vi "_PC_Daemon_Laser_CheckEmission.vi"(1 "stopRefnum":refnum<vi>, 2 "error in (no error)":errorcluster, 3 "LaserSetting":T1={"Energy"=50.0, "Freq"=100.0, "Emission"=FALSE, "TriggerSource"=enum."Internal", "Time Stamp"=timestamp(0 s since 1904-01-01)}) -> (0 "error out":errorcluster)   [LabVIEW 2018]
uses:
  RT/ControlLoop/Laser/Ctl/_ctl_LaserParam.ctl
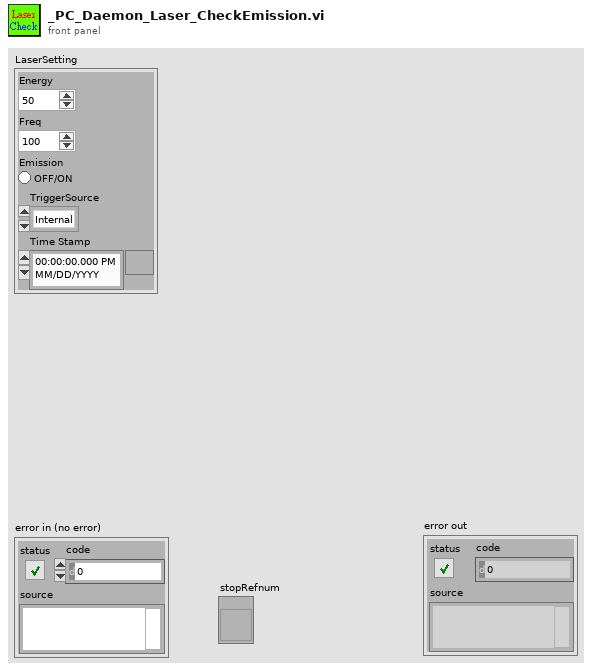
[diagram p1: front panel]
types:
  T1 = typedef "_ctl_LaserParam.ctl" = cluster{"Energy":dbl, "Freq":dbl, "Emission":bool, "TriggerSource":enum16{"Internal", "External"}, "Time Stamp":timestamp}
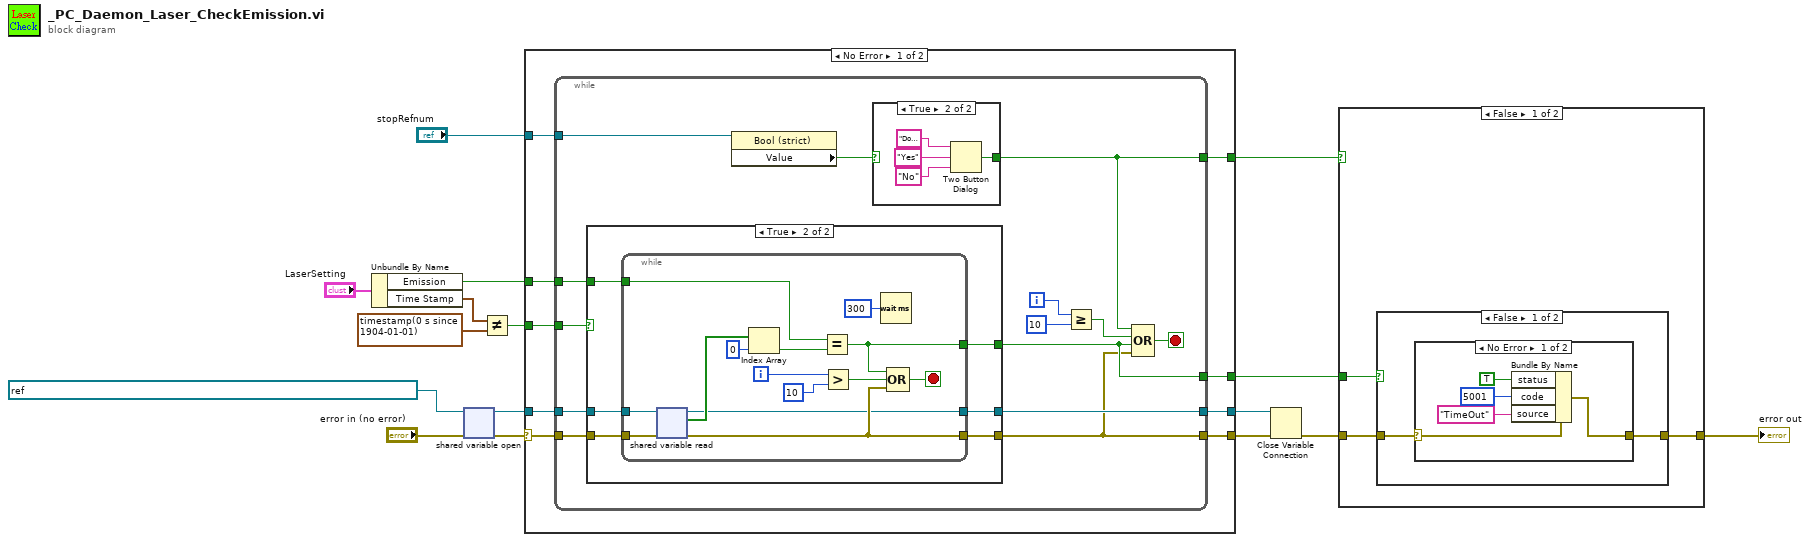
[diagram p0: block diagram]
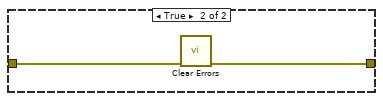
[diagram p4: hidden frame]
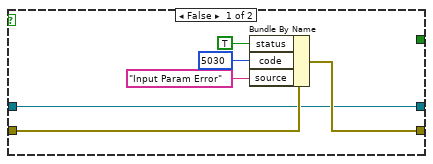
[diagram p6: hidden frame]
diagram:
  n1 = Unbundle By Name("LaserSetting") -> ("Emission"=w14:bool, "Time Stamp"=w16:timestamp)
  n2 = shared-variable-open(refnum<k21> "ni.var.psp://NI-sbRIO/_RT_CtrlLoop_Laser_Variables/LaserStatusByte" ("shared variable refnum in"), "error in (no error)") -> (w7:refnum<k21>, w6:errorcluster)
  n3 = Not Equal?(x=w16, y=timestamp(0 s since 1904-01-01)) -> (x != y?=w13:bool)
  n4 = case shown="No Error" w6 {
    selector: w6 -> [w20 w72]
    tunnel: w14 -> [w25 _]
    tunnel: w13 -> [w24 _]
    tunnel: [w23 w72] -> w4
    tunnel: [w22 _] -> w11
    tunnel: w7 -> [w21 w71]
    tunnel: [w19 w71] -> w5
    tunnel: "stopRefnum" -> [w18 _]
    tunnel: [w17 _] -> w1
    frame No Error {
      n5 = while {
        tunnel: w25 -> [w39]
        tunnel: w24 -> [w38]
        tunnel: [w29] -> w23
        tunnel: [w33] -> w22
        tunnel: w21 -> [w32]
        tunnel: w20 -> [w31]
        tunnel: [w30] -> w19
        tunnel: w18 -> [w28]
        tunnel: [w26] -> w17
        i -> [w37]
        stop <- w34 stop-if-true
        n6 = case shown="True" w38 {
          tunnel: w39 -> [_ w56]
          tunnel: [_ w55] -> w33
          tunnel: w32 -> [w45 w54]
          tunnel: w31 -> [w47 w53]
          tunnel: [w46 w52] -> w29
          tunnel: [w45 w51] -> w30
          frame False {
            n7 = Bundle By Name(cluster=w47, "status"=TRUE, "code"=5030, "source"="Input Param Error") -> (w46:errorcluster)
          }
          frame True {
            n8 = while {
              tunnel: w56 -> [w66]
              tunnel: [w63] -> w55
              tunnel: w54 -> [w62]
              tunnel: w53 -> [w61]
              tunnel: [w58] -> w52
              tunnel: [w57] -> w51
              i -> [w65]
              stop <- w67 stop-if-true
              n9 = shared-variable-read(w62, w61) -> (w57:refnum<k21>, w58:errorcluster, w60:bool[])
              n10 = Index Array(array=w60, index=0) -> (element=w69:bool)
              n11 = Equal?(x=w66, y=w69) -> (x = y?=w63:bool)
              n12 = Greater?(x=w65, y=10) -> (0:w59:bool)
              n13 = Wait (ms)(milliseconds to wait=u32 300) -> ()  [unwired: 1 out]
              n14 = Compound Arithmetic op=OR(w63, w59, w58) -> (w67:bool)
            }
          }
        }
        n15 = property class="Bool (strict)"(reference=w28) -> ("Value"=w27:bool)  [unwired: 1 in, 2 out]
        n16 = case shown="True" w27 {
          selector: w27 -> [w40 _]
          tunnel: [w40 w41] -> w26
          frame False {
          }
          frame True {
            n17 = Two Button Dialog(message="Do you want to confirm the interrupt in the parameter setting?", 1:"No" ("F button name (\"Cancel\")"), 2:"Yes" ("T button name (\"OK\")")) -> (T button?=w41:bool)
          }
        }
        n18 = Greater Or Equal?(x=w37, y=10) -> (x >= y?=w35:bool)
        n19 = Compound Arithmetic op=OR(w26, w35, w33, w29) -> (w34:bool)
      }
    }
    frame Error {
    }
  }
  n20 = Close Variable Connection(8:w4, 11:w5) -> (0:w3:errorcluster)
  n21 = case shown="False" w1 {
    tunnel: w11 -> [w75 _]
    tunnel: [w74 w85] -> w10
    tunnel: w3 -> [w73 w86]
    frame False {
      n22 = case shown="False" w75 {
        tunnel: w73 -> [w77 w84]
        tunnel: [w76 w84] -> w74
        frame False {
          n23 = case shown="No Error" w77 {
            selector: w77 -> [w79 w83]
            tunnel: [w78 w83] -> w76
            frame No Error {
              n24 = Bundle By Name(cluster=w79, "status"=TRUE, "code"=5001, "source"="TimeOut") -> (w78:errorcluster)
            }
            frame Error {
            }
          }
        }
        frame True {
        }
      }
    }
    frame True {
      n25 = call <vilib>:"Clear Errors.vi"("error in (no error)"=w86) -> ("error out"=w85:errorcluster)  [unwired: 5 in, 1 out]
    }
  }
  "error out" <- w10
